vi "Refresh Layout From VI.vi"(8 "error in":errorcluster, 10 "VI refnum":refnum<vi>, 11 "VI Panel Layout in":refnum<class "VI Panel Layout.lvclass">) -> (0 "error out":errorcluster, 3 "VI Panel Layout out":refnum<class "VI Panel Layout.lvclass">, 4 "subpanel refnums":refnum<vi>[](array[refnum]), 6 "subpanel UIDs":i32[](array[numeric]))   [LabVIEW 2012, in "NI_SE_Front Panel Layout.lvlib" / "VI Panel Layout.lvclass"]
uses:
  VI Panel Layout.lvclass
  Object Layout Classes/Object Layout/Object Layout.lvclass
  Object Layout Classes/Object Layout/Object Layout.lvclass/Object Layout.ctl
  VI Panel Layout.lvclass/VI Panel Layout.ctl
  Subpanel VI Pair.ctl
  Object Layout Classes/Object Layout/Get UID.vi
  Object Layout Classes/Object Layout/Get Unique Name.vi
  Convert UID To String.vi
  NI_SE_Front Panel Layout.lvlib
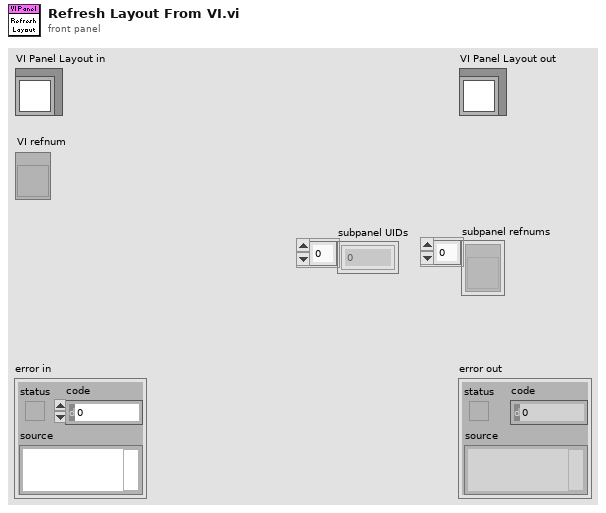
[diagram p1: front panel]
types:
  T1 = typedef "NI_SE_Front Panel Layout.lvlib/VI Panel Layout.lvclass/Subpanel VI Pair.ctl" = cluster{"subpanel UID":i32, "VI name":string, "VI path (rel)":path}
  T2 = typedef "LVRectTypeDef.ctl" = cluster{"Left":i16, "Top":i16, "Right":i16, "Bottom":i16}
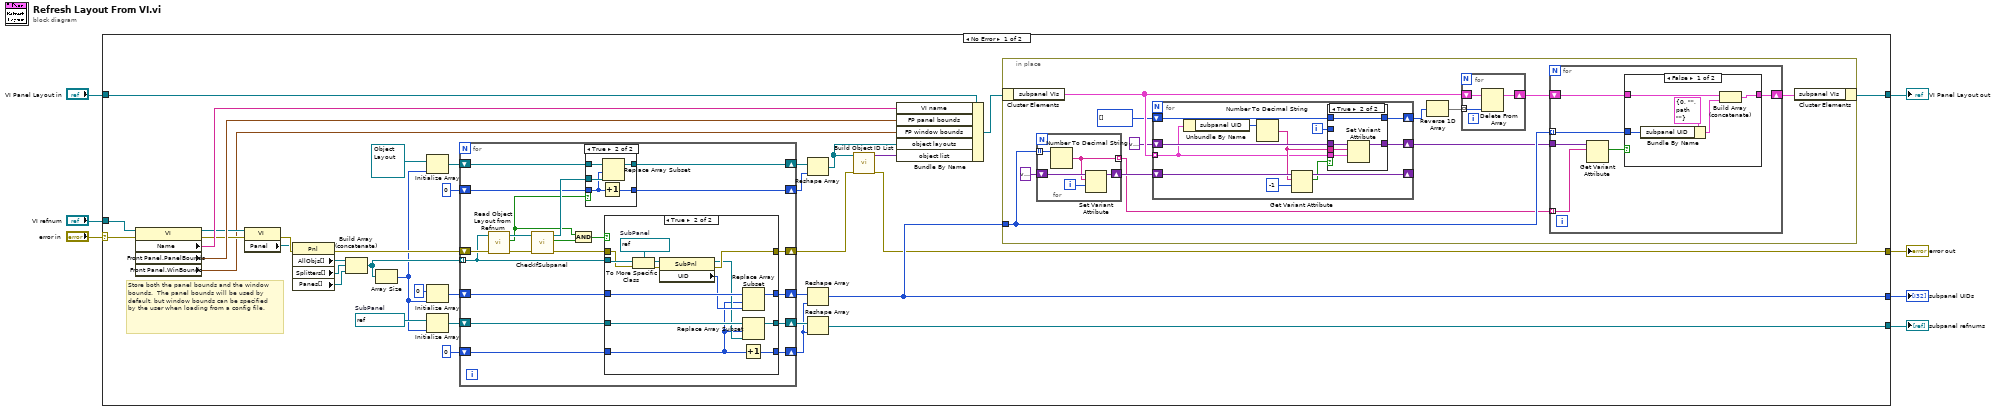
[diagram p0: block diagram]
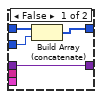
[diagram p3: hidden frame]
diagram:
  n1 = case shown="No Error" "error in" {
    selector: "error in" -> [w34 w144]
    tunnel: [w8 w144] -> w6
    tunnel: [w31 w143] -> w4
    tunnel: "VI Panel Layout in" -> [w33 w143]
    tunnel: "VI refnum" -> [w35 _]
    tunnel: [w16 _] -> w2
    tunnel: [w18 _] -> w1
    frame No Error {
      w14 = refnum<vi> refnum  # SubPanel
      # "Store both the panel bounds and the window bounds.  The panel bounds will be used by default, but window bounds can be specified by the user when loading from a config file."
      n2 = property class="VI"(reference=w35, error in=w34) -> (reference out=w41:refnum<vi>, error out=w42:errorcluster, "Name"=w43:string, "Front Panel.PanelBounds"=w44:T2, "Front Panel.WinBounds"=w29:T2)
      n3 = property class="VI"(reference=w41, error in=w42) -> (error out=w37:errorcluster, "Panel"=w36:refnum<vi>)  [unwired: 1 out]
      n4 = property class="Pnl"(reference=w36, error in=w37) -> (error out=w38:errorcluster, "AllObjs[]"=w40:refnum<vi>[], "Splitters[]"=w39:refnum<vi>[], "Panes[]"=w30:refnum<vi>[])  [unwired: 1 out]
      n5 = Build Array (concatenate)(w40, w39, w30) -> (w27:refnum<vi>[])
      n6 = Array Size(array=w27) -> (size(s)=w12:i32)
      n7 = Initialize Array(refnum<class "Object Layout.lvclass"> refnum ("Object Layout out"), w12) -> (w26:refnum<class "Object Layout.lvclass">[])
      n8 = Initialize Array(0 ("UID"), w12) -> (w21:i32[])
      n9 = Initialize Array(w14, w12) -> (w13:refnum<vi>[])
      n10 = for {
        tunnel: w27 -> [w112] mode=indexing
        shift-right: [w111] -> w9
        shift-left: w38 -> [w117]
        shift-right: [w106] -> w24
        shift-left: w26 -> [w107]
        shift-right: [w103] -> w19
        shift-left: w21 -> [w105]
        shift-right: [w102] -> w17
        shift-left: w13 -> [w104]
        shift-right: [w100] -> w23
        shift-left: 0 -> [w101]
        shift-right: [w98] -> w15
        shift-left: 0 -> [w99]
        n11 = call "Read Object Layout from Refnum.vi"("error in"=w117, "GObj refnum"=w112) -> ("error out"=w114:errorcluster, "found?"=w110:bool, "object layout"=w116:refnum<class "Object Layout.lvclass">)  [unwired: 7 in]
        n12 = call-dynamic "CheckIfSubpanel.vi"("error in"=w114, "Object Layout in"=w116) -> ("error out"=w113:errorcluster, "subpanel?"=w109:bool, "Object Layout out"=w115:refnum<class "Object Layout.lvclass">)  [unwired: 7 in]
        n13 = And(x=w110, y=w109) -> (x .and. y?=w108:bool)
        n14 = case shown="True" w110 {
          tunnel: w107 -> [w119 w124]
          tunnel: w115 -> [_ w122]
          tunnel: [w119 w123] -> w106
          tunnel: w101 -> [w118 w121]
          tunnel: [w118 w120] -> w100
          frame False {
          }
          frame True {
            n15 = Increment(x=w121) -> (x+1=w120:i32)
            n16 = Replace Array Subset(array=w124, new element=w122, index=w121) -> (w123:refnum<class "Object Layout.lvclass">[])
          }
        }
        n17 = case shown="True" w108 {
          tunnel: w113 -> [w128 w139]
          tunnel: w112 -> [_ w141]
          tunnel: [w128 w142] -> w111
          tunnel: w105 -> [w127 w135]
          tunnel: [w127 w134] -> w103
          tunnel: w104 -> [w126 w132]
          tunnel: [w126 w131] -> w102
          tunnel: w99 -> [w125 w129]
          tunnel: [w125 w136] -> w98
          frame False {
          }
          frame True {
            w137 = refnum<vi> refnum  # SubPanel
            n18 = To More Specific Class(target class=w137, reference=w141, error in=w139) -> (specific class reference=w140:refnum<vi>, error out=w138:errorcluster)
            n19 = property class="SubPnl"(reference=w140, error in=w138) -> (reference out=w130:refnum<vi>, error out=w142:errorcluster, "UID"=w133:i32)
            n20 = Replace Array Subset(array=w135, new element=w133, index=w129) -> (w134:i32[])
            n21 = Replace Array Subset(array=w132, new element=w130, index=w129) -> (w131:refnum<vi>[])
            n22 = Increment(x=w129) -> (x+1=w136:i32)
          }
        }
      }
      n23 = Reshape Array(w24, w23) -> (w10:refnum<class "Object Layout.lvclass">[])
      n24 = Reshape Array(w19, w15) -> (w18:i32[])
      n25 = Reshape Array(w17, w15) -> (w16:refnum<vi>[])
      n26 = call "Build Object ID List.vi"("error in"=w9, "object layouts"=w10) -> ("error out"=w8:errorcluster, "object ID list"=w11:variant)  [unwired: 8 in]
      n27 = Bundle By Name(cluster=w33, "VI name"=w43, "FP panel bounds"=w44, "FP window bounds"=w29, "object layouts"=w10, "object list"=w11) -> (w32:refnum<class "VI Panel Layout.lvclass">)
      n28 = in-place {
        in-place-border: w18 -> [w50]
        n29 = in-place-cluster #1(w32) -> ("subpanel VIs"=w54:T1[])
        n30 = for {
          shift-right: [w97] -> w55
          shift-left: variant -> [w96]
          tunnel: w50 -> [w94] mode=indexing
          tunnel: [w93] -> w45 mode=indexing
          i -> [w95]
          n31 = Number To Decimal String(number=w94) -> (decimal integer string=w93:string)  [unwired: 1 in]
          n32 = Set Variant Attribute(Variant=w96, name=w93, value=w95) -> (Variant out=w97:variant)  [unwired: 1 in, 2 out]
        }
        n33 = for {
          tunnel: w54 -> [w75] mode=indexing
          shift-right: [w80] -> _
          shift-left: w55 -> [w82]
          shift-right: [w78] -> w47
          shift-left: variant -> [w77]
          shift-right: [w72] -> w53
          shift-left: i32[] [] ("Array") -> [w74]
          i -> [w73]
          n34 = Unbundle By Name(w75) -> ("subpanel UID"=w83:i32)
          n35 = Number To Decimal String(number=w83) -> (decimal integer string=w76:string)  [unwired: 1 in]
          n36 = Get Variant Attribute(Variant=w82, name=w76, default value (empty Variant)=-1) -> (duplicate Variant=w80:variant, found=w79:bool)  [unwired: 1 in, 2 out]
          n37 = case shown="True" w79 {
            tunnel: [w87 w92] -> w78
            tunnel: w77 -> [w87 w91]
            tunnel: w76 -> [_ w90]
            tunnel: w75 -> [_ w89]
            tunnel: w74 -> [w86 w88]
            tunnel: [w85 w88] -> w72
            tunnel: w73 -> [w84 _]
            frame False {
              n38 = Build Array (concatenate)(w86, w84) -> (w85:i32[])
            }
            frame True {
              n39 = Set Variant Attribute(Variant=w91, name=w90, value=w89) -> (Variant out=w92:variant)  [unwired: 1 in, 2 out]
            }
          }
        }
        n40 = Reverse 1D Array(array=w53) -> (reversed array=w52:i32[])
        n41 = for {
          shift-right: [w70] -> w49
          shift-left: w54 -> [w71]
          tunnel: w52 -> [w69] mode=indexing
          n42 = Delete From Array(array=w71, index=w69) -> (array with subset deleted=w70:T1[])  [unwired: 1 in, 1 out]
        }
        n43 = for {
          tunnel: w50 -> [w58] mode=indexing
          shift-right: [w59] -> w48
          shift-left: w49 -> [w60]
          tunnel: w47 -> [w62]
          tunnel: w45 -> [w57] mode=indexing
          n44 = Get Variant Attribute(Variant=w62, name=w57) -> (found=w61:bool)  [unwired: 2 in, 3 out]
          n45 = case shown="False" w61 {
            tunnel: w60 -> [w67 w68]
            tunnel: [w66 w68] -> w59
            tunnel: w58 -> [w64 _]
            frame False {
              n46 = Bundle By Name(cluster=T1 {"subpanel UID"=0, "VI name"="", "VI path (rel)"=path ""} ("subpanel VI pair"), "subpanel UID"=w64) -> (w63:T1)
              n47 = Build Array (concatenate)(w67, w63) -> (w66:T1[])
            }
            frame True {
            }
          }
        }
        n48 = in-place-cluster #1("subpanel VIs"=w48) -> (w31:refnum<class "VI Panel Layout.lvclass">)
      }
    }
    frame Error {
    }
  }
  "error out" <- w6
  "VI Panel Layout out" <- w4
  "subpanel refnums" <- w2
  "subpanel UIDs" <- w1
